vi "Module Type.vi"(11 "Triggered Logger in":refnum<class "Triggered Logger.lvclass">) -> (2 "Module Type":string)   [LabVIEW 2020, in "VolatusData.lvlib" / "Triggered Logger.lvclass"]
uses:
  Triggered Logger.lvclass
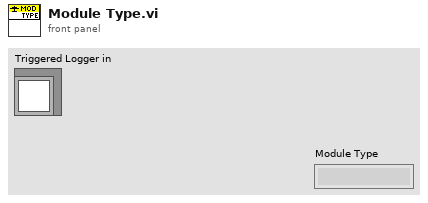
[diagram p1: front panel]
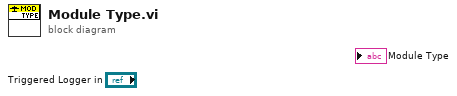
[diagram p0: block diagram]
diagram:
